vi "SE_HV500.ProcDestructor.vi"(0 "i ref in":refnum<vi>, 3 "ms timeout (100)":i32=100, 5 "error in (no error)":errorcluster) -> (14 "i ref out":refnum<vi>, 17 "timed out":bool, 19 "error out":errorcluster)   [LabVIEW 2014, in "SE_HV500.lvlib"]
doc: "This is the counterpart to ProcConstructor and is called befor the \"deactivate\" is called. This can be used to shutdown/deinitialize things."
uses:
  SE_HV500.lvlib
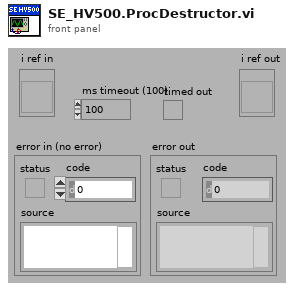
[diagram p1: front panel]
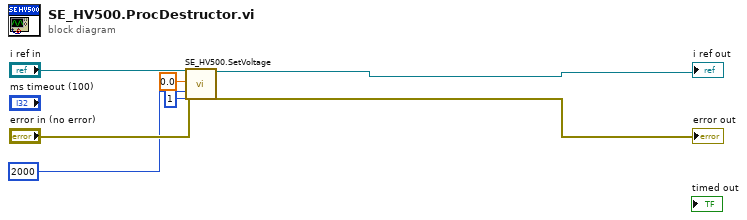
[diagram p0: block diagram]
diagram:
  n1 = call "SE_HV500.SetVoltage.vi"("i ref in"="i ref in", "Set Voltage"=0.0, "Channel"=i16 1, "Time out"=2000, "error in (no error)"="error in (no error)") -> ("i ref out"=→"i ref out":refnum<vi>, "error out"=→"error out":errorcluster)  [unwired: 12 in, 1 out]
